vi "Construct LNA.vi"(8 "error in (no error)":errorcluster, 10 "Client GUID":string) -> (0 "error out":errorcluster, 3 "Client Proxy LNA out":refnum<class "Client Proxy LNA.lvclass">)   [LabVIEW 2016, in "Client Proxy LNA.lvlib" / "Client Proxy LNA.lvclass"]
doc: "Creates a new instance of the LNA\nthat will send commands to and from\nthe client. This constructor stores the\nuser visible name, GUID, IP address, \ntimeout and buffer size and returns the \nLNA object"
uses:
  Client Proxy LNA.lvclass
  C:/Program Files (x86)/National Instruments/LabVIEW 2016/vi.lib/NI/Actors/Linked Network Actor/Linked Network Actor/Linked Network Actor.lvclass
  <vilib>/NI/Actors/Linked Network Actor/Linked Network Actor/Linked Network Actor.lvclass
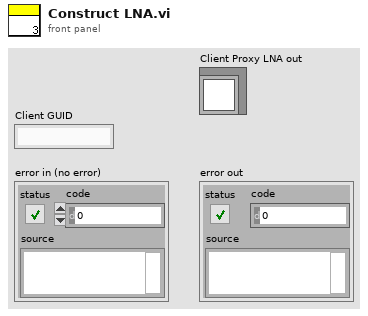
[diagram p1: front panel]
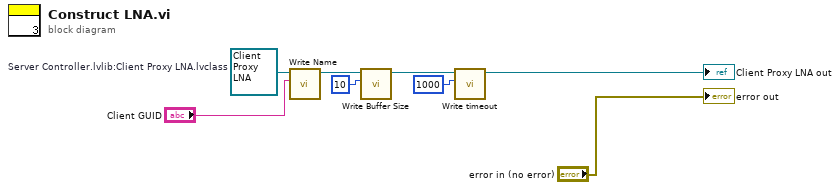
[diagram p0: block diagram]
diagram:
  w5 = refnum<class "Client Proxy LNA.lvclass"> refnum  # Server Controller.lvlib:Client Proxy LNA.lvclass
  n1 = call <vilib>:"Write Name.vi"("Name"="Client GUID", "Network Actor in"=w5) -> ("Network Actor out"=w1:refnum<class "Client Proxy LNA.lvclass">)  [unwired: 9 in]
  n2 = call <vilib>:"Write Buffer Size.vi"("Buffer Size"=10, "Network Actor in"=w1) -> ("Network Actor out"=w2:refnum<class "Client Proxy LNA.lvclass">)  [unwired: 9 in]
  n3 = call <vilib>:"Write timeout.vi"("timeout"=1000, "Network Actor in"=w2) -> ("Network Actor out"=→"Client Proxy LNA out":refnum<class "Client Proxy LNA.lvclass">)  [unwired: 9 in]
  "error out" <- "error in (no error)"
